vi "Router - Create Master Table.vi"(8 "error in (no error)":errorcluster, 11 "Router Data In":T1) -> (0 "error out":errorcluster, 3 "Router Data Out":T1)   [LabVIEW 2016, in "PXImc Router.lvlib"]
uses:
  PXImc Router.lvlib
  Controls/Router - Configuration.ctl
  Controls/Target Type.ctl
  Controls/Router/Node Block R-W Properties.ctl
  Controls/Router/Block Properties.ctl
  Controls/Router/Router - PXImc Properties.ctl
  Controls/Router/Router - PXImc Card Properties.ctl
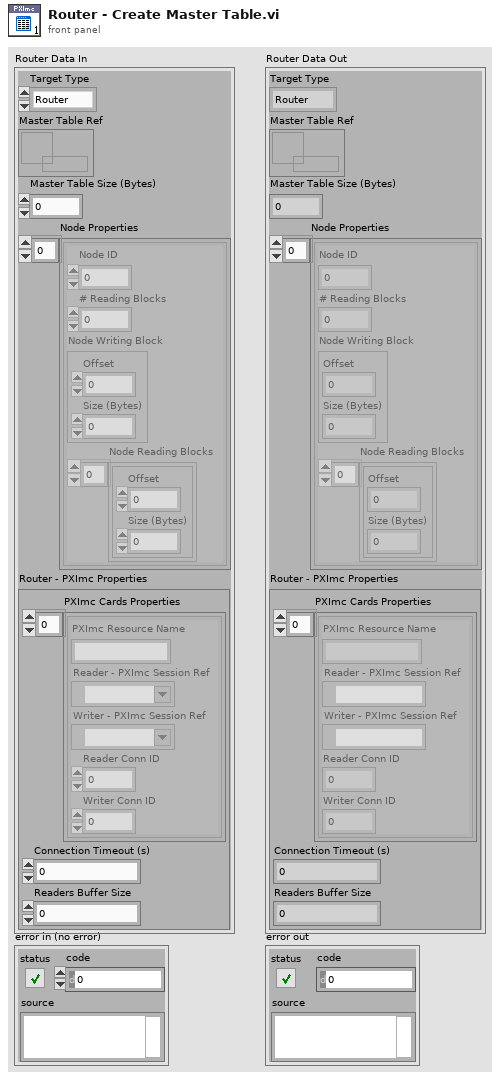
[diagram p1: front panel]
types:
  T1 = typedef "PXImc Router.lvlib/Router - Configuration.ctl" = cluster{"Target Type":T2, "Master Table Ref":refnum<data-value>, "Master Table Size (Bytes)":u32, "Node Properties":T3[], "Router - PXImc Properties":T5}
  T2 = typedef "PXImc Router.lvlib/Target Type.ctl" = enum16{"Router", "Node"}
  T3 = typedef "PXImc Router.lvlib/Node Block R-W Properties.ctl" = cluster{"Node ID":u32, "# Reading Blocks":u32, "Node Writing Block":T4, "Node Reading Blocks":T4[]}
  T4 = typedef "PXImc Router.lvlib/Block Properties.ctl" = cluster{"Offset":u32, "Size (Bytes)":u32}
  T5 = typedef "PXImc Router.lvlib/Router - PXImc Properties.ctl" = cluster{"PXImc Cards Properties":T6[], "Connection Timeout (s)":dbl, "Readers Buffer Size":u64}
  T6 = typedef "PXImc Router.lvlib/Router - PXImc Card Properties.ctl" = cluster{"PXImc Resource Name":string, "Reader - PXImc Session Ref":refnum<k21>, "Writer - PXImc Session Ref":refnum<k21>, "Reader Conn ID":u16, "Writer Conn ID":u16}
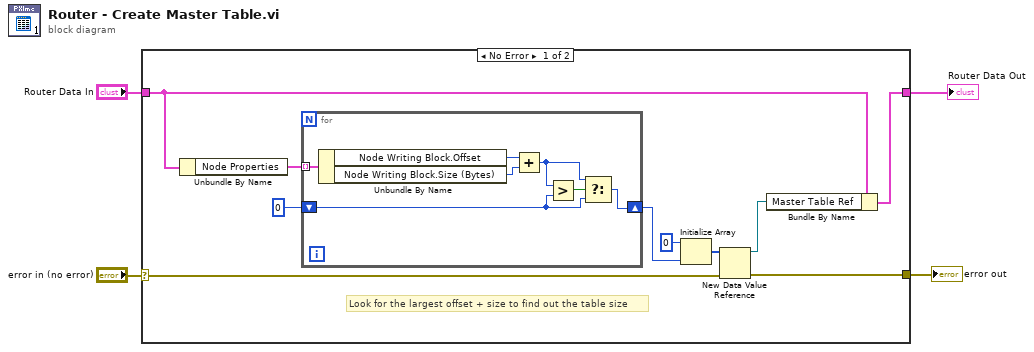
[diagram p0: block diagram]
diagram:
  n1 = case shown="No Error" "error in (no error)" {
    selector: "error in (no error)" -> [w6 w22]
    tunnel: [w14 w23] -> w4
    tunnel: "Router Data In" -> [w13 w23]
    tunnel: [w8 w22] -> w2
    frame No Error {
      # "Look for the largest offset + size to find out the table size"
      n2 = Unbundle By Name(w13) -> ("Node Properties"=w11:T3[])
      n3 = for {
        tunnel: w11 -> [w21] mode=indexing
        shift-right: [w15] -> w5
        shift-left: u32 0 ("Offset") -> [w16]
        n4 = Unbundle By Name(w21) -> ("Node Writing Block.Offset"=w20:u32, "Node Writing Block.Size (Bytes)"=w19:u32)
        n5 = Add(x=w20, y=w19) -> (x+y=w17:u32)
        n6 = Greater?(x=w17, y=w16) -> (0:w18:bool)
        n7 = Select(t=w17, s=w18, f=w16) -> (s? t:f=w15:u32)
      }
      n8 = Initialize Array(u8 0 ("element"), w5) -> (w10:u8[])
      n9 = New Data Value Reference(data value=w10, error in=w6) -> (data value reference=w7:refnum<data-value>, error out=w8:errorcluster)
      n10 = Bundle By Name(cluster=w13, "Master Table Ref"=w7) -> (w14:T1)
    }
    frame Error {
    }
  }
  "Router Data Out" <- w4
  "error out" <- w2
